vi "SETID.vi"() -> ()   [LabVIEW 2016]
uses:
  Classes/BML_Frame_SetID/BML_Frame_SetID.lvclass
  C:/Users/8135/Desktop/BML_Pattern_Gen/BeamLink_Pattern_Gen/BML_Pattern_Gen_Refactor/Classes/BML_Frame_Root/BML_Frame_Root.lvclass
  Classes/BML_DigiPattern_Generator/DigiPattern_Generator.lvclass
  Classes/Config_Read/Frame_Data.ctl
  Classes/Config_Read/OperationMode.ctl
  Classes/Config_Read/BurstLength.ctl
  Classes/Config_Read/RW_Option.ctl
  Classes/BML_Frame_RW/BML_Frame_RW.lvclass
  Classes/Config_Read/Config_Read_BML.lvclass
panel:
  out "error out":errorcluster
  in  "PinMap":path
  in  "ChipID":u8=1
  in  "Config Path":path
  in  "error in (no error)":errorcluster
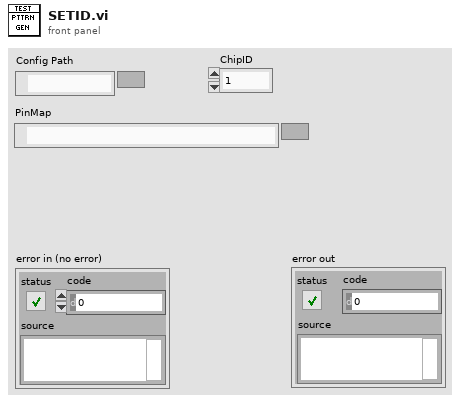
[diagram p1: front panel]
types:
  T1 = typedef "Config_Read_BML.lvclass/Frame_Data.ctl" = cluster{"Pattern_Name":string, "Operation Mode":T2, "BurstLength":T3, "FSN":u8, "Start_Addr":u16, "Data":u8[], "R/W?":T4, "Opcode":string[], "ChipID":u8}
  T2 = typedef "Config_Read_BML.lvclass/OperationMode.ctl" = enum8{"Normal", "ImmeEffect", "InitSlaveID", "LoadData"}
  T3 = typedef "Config_Read_BML.lvclass/BurstLength.ctl" = enum8{"0", "2", "3", "4", "5", "8", "16", "32"}
  T4 = typedef "Config_Read_BML.lvclass/RW_Option.ctl" = enum16{"Read", "Write", "R/W"}
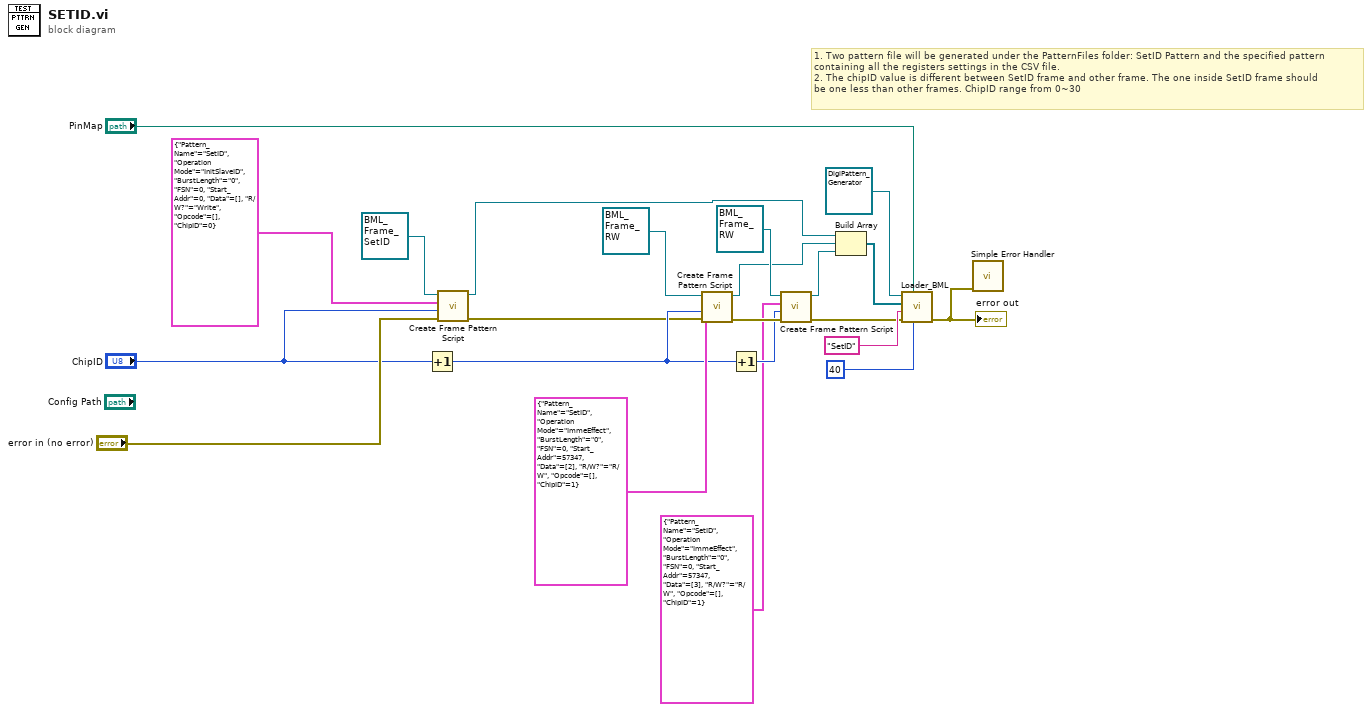
[diagram p0: block diagram]
diagram:
  # "1. Two pattern file will be generated under the PatternFiles folder: SetID Pattern and the specified pattern\ncontaining all the registers settings in the CSV file.\n2. The chipID value is different between SetID frame and other frame. The one inside SetID frame should \nbe one less than other frames. ChipID range from 0~30"
  n1 = Increment(x="ChipID") -> (x+1=w9:u8)
  n2 = call-dynamic "Create Frame Pattern Script.vi"("error in (no error)"="error in (no error)", "ChipID"="ChipID", "Frame_Data"=T1 {"Pattern_Name"="SetID", "Operation Mode"=enum."InitSlaveID", "BurstLength"=enum."0", "FSN"=0, "Start_Addr"=0, "Data"=[], "R/W?"=enum."Write", "Opcode"=[], "ChipID"=0}, "BML_Frame_SetID in"=refnum<class "BML_Frame_SetID.lvclass"> refnum ("BML_Frame_SetID.lvclass")) -> ("error out"=w1:errorcluster, "BML_Frame_SetID out"=w5:refnum<class "BML_Frame_SetID.lvclass">)  [unwired: 6 in]
  n3 = call-dynamic "Create Frame Pattern Script.vi"("error in (no error)"=w1, "ChipID"=w9, "Frame_Data"=T1 {"Pattern_Name"="SetID", "Operation Mode"=enum."ImmeEffect", "BurstLength"=enum."0", "FSN"=0, "Start_Addr"=57347, "Data"=[2], "R/W?"=enum."R/W", "Opcode"=[], "ChipID"=1}, "BML_Frame_RW in"=refnum<class "BML_Frame_RW.lvclass"> refnum ("BML_Frame_RW.lvclass")) -> ("error out"=w10:errorcluster, "BML_Frame_RW out"=w4:refnum<class "BML_Frame_RW.lvclass">)  [unwired: 6 in]
  n4 = Increment(x=w9) -> (x+1=w8:u8)
  n5 = call-dynamic "Create Frame Pattern Script.vi"("error in (no error)"=w10, "ChipID"=w8, "Frame_Data"=T1 {"Pattern_Name"="SetID", "Operation Mode"=enum."ImmeEffect", "BurstLength"=enum."0", "FSN"=0, "Start_Addr"=57347, "Data"=[3], "R/W?"=enum."R/W", "Opcode"=[], "ChipID"=1}, "BML_Frame_RW in"=refnum<class "BML_Frame_RW.lvclass"> refnum ("BML_Frame_RW.lvclass")) -> ("error out"=w6:errorcluster, "BML_Frame_RW out"=w3:refnum<class "BML_Frame_RW.lvclass">)  [unwired: 6 in]
  n6 = Build Array(w5, w4, w3) -> (w2:refnum<class "BML_Frame_Root.lvclass">[])
  n7 = call "Loader_BML.vi"("Timeset between frms"=u32 40, "PinMap"="PinMap", "error in (no error)"=w6, "Pattern Name"="SetID", "BML Frame Array"=w2, "BML_DigiPattern_Generator.lvclass"=refnum<class "DigiPattern_Generator.lvclass"> refnum) -> ("error out"=w17:errorcluster)  [unwired: 4 in, 1 out]
  "error out" <- w17
  n8 = call <vilib>:"Simple Error Handler.vi"("error in (no error)"=w17) -> ()  [unwired: 4 in, 5 out]
